vi "test_FXP16.5 Write and Read_Lower Than Minimum.vi"(8 "error in (no error)":errorcluster, 11 "Scalar Channels Testing in":refnum<class "FPGA Addon Scalar Channels System Tests.lvclass">=refnum) -> (0 "error out":errorcluster, 3 "Scalar Channels Testing out":refnum<class "FPGA Addon Scalar Channels System Tests.lvclass">)   [LabVIEW 2019, in "FPGA Addon Scalar Channels System Tests.lvclass"]
uses:
  FPGA Addon Scalar Channels System Tests.lvclass
  FPGA Addon Test Class/FPGA Addon Test Class.lvclass
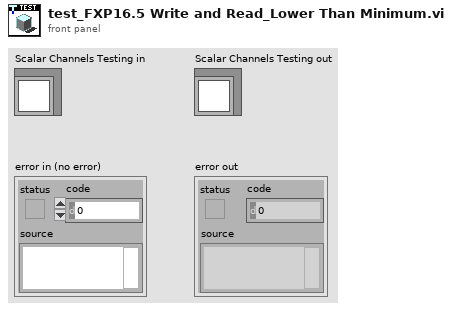
[diagram p1: front panel]
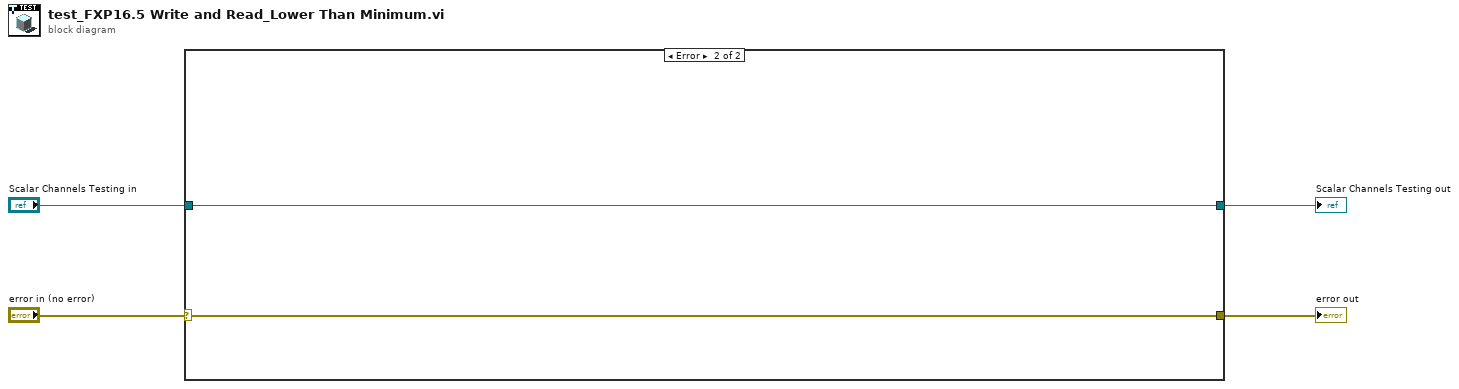
[diagram p0: block diagram]
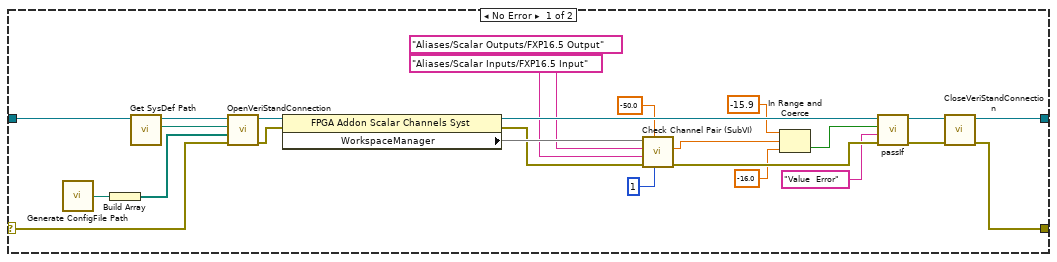
[diagram p2: hidden frame]
diagram:
  n1 = case shown="Error" "error in (no error)" {
    selector: "error in (no error)" -> [w22 w31]
    tunnel: [w28 w31] -> w3
    tunnel: [w29 w30] -> w1
    tunnel: "Scalar Channels Testing in" -> [w21 w30]
    frame No Error {
      n2 = call "Generate ConfigFile Path.vi"() -> ("ConfigFile path"=w12:path)
      n3 = Build Array(w12) -> (w11:path[])
      n4 = call "Get SysDef Path.vi"("Scalar Channels Testing in"=w21) -> ("SysDef Path"=w19:path, "Scalar Channels Testing out"=w20:refnum<class "FPGA Addon Test Class.lvclass">)  [unwired: 9 in]
      n5 = call-dynamic "OpenVeriStandConnection.vi"("error in (no error)"=w22, "overrides files"=w11, "System Definition File"=w19, "VeriStand Test Case in"=w20) -> ("error out"=w27:errorcluster, "VeriStand Test Case out"=w26:refnum<class "FPGA Addon Scalar Channels System Tests.lvclass">)  [unwired: 5 in, 1 out]
      n6 = property class="FPGA Addon Scalar Channels Syst"(reference=w26, error in=w27) -> (reference out=w25:refnum<class "FPGA Addon Scalar Channels System Tests.lvclass">, error out=w15:errorcluster, "WorkspaceManager"=w18)
      n7 = call "Check Channel Pair (SubVI).vi"("seconds to wait"=u32 1 ("milliseconds to wait"), "OutputChannel Value in"=-50.0 ("Value"), "error in (no error)"=w15, "Input Channel"="Aliases/Scalar Inputs/FXP16.5 Input" ("Channel"), "Output Channel"="Aliases/Scalar Outputs/FXP16.5 Output" ("Channel"), "WorkspaceManager in"=w18) -> ("error out"=w16:errorcluster, "InputChanel Value"=w9:dbl)  [unwired: 2 in, 2 out]
      n8 = In Range and Coerce(upper limit=-15.9 ("Value"), x=w9, lower limit=-16.0 ("Value")) -> (In Range?=w8:bool)  [unwired: 1 out]
      n9 = call-dynamic "passIf.vi"("error in (no error)"=w16, "message (\"\")"="Value  Error" ("message (\"\")"), "pass"=w8, "TestCase in"=w25) -> ("error out"=w23:errorcluster, "TestCase out"=w24:refnum<class "FPGA Addon Scalar Channels System Tests.lvclass">)  [unwired: 6 in]
      n10 = call-dynamic "CloseVeriStandConnection.vi"("error in (no error)"=w23, "VeriStand Test Case in"=w24) -> ("error out"=w28:errorcluster, "VeriStand Test Case out"=w29:refnum<class "FPGA Addon Scalar Channels System Tests.lvclass">)  [unwired: 8 in]
    }
    frame Error {
    }
  }
  "error out" <- w3
  "Scalar Channels Testing out" <- w1
